vi "FileTrcOpen.vi"(6 "提示语":refnum<vi>, 7 "Language":u32, 8 "进度条":refnum<vi>, 9 "进度数值":refnum<vi>, 10 "报文行数统计":refnum<vi>, 11 "file path (dialog if empty)":path caption="文件路径 （空时为对话框）") -> (0 "路径输出":path, 1 "重构的Data数组":u32[][](array[numeric]), 2 "统计数量":string[](array[string]), 3 "报文ID":string[](array[string]), 4 "基时间簇":T1 {"基时间秒" format="%#.6f"}, 5 "CAN报文统计":string[][](array[string]))   [LabVIEW 2015]
uses:
  <vilib>/Utility/file.llb/Read Delimited Spreadsheet (string).vi
  <vilib>/regexp/Match Regular Expression.xnode
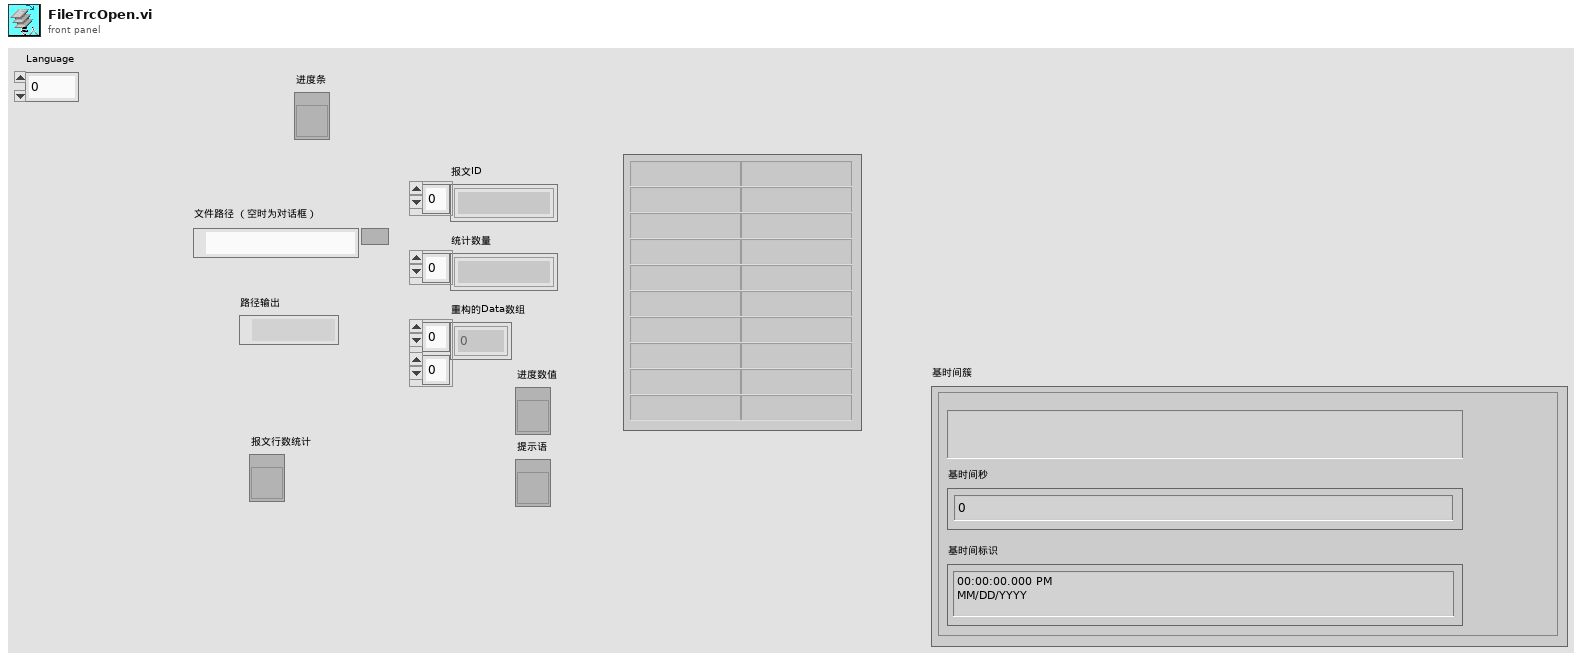
[diagram p1: front panel]
types:
  T1 = cluster{"基时间字符串":string, "基时间秒":dbl, "基时间标识":timestamp}
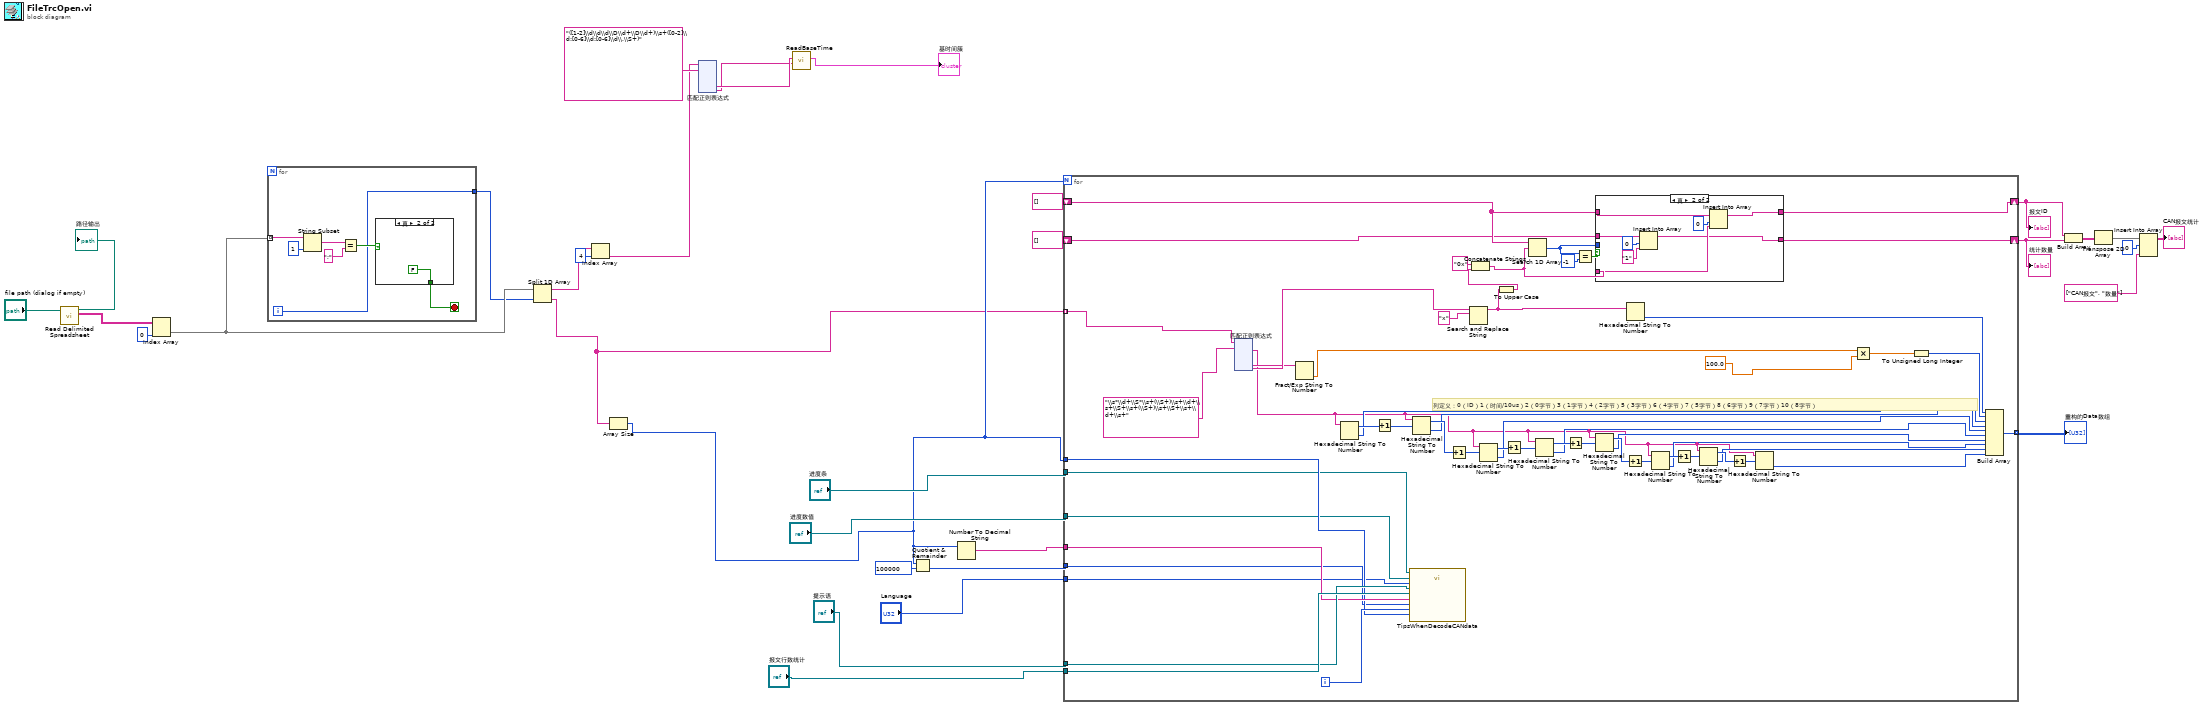
[diagram p0: block diagram]
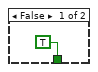
[diagram p2: hidden frame]
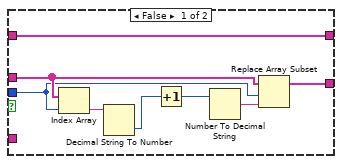
[diagram p3: hidden frame]
diagram:
  n1 = call-poly <vilib>:"Read Delimited Spreadsheet.vi"("file path (dialog if empty)"="file path (dialog if empty)") -> ("new file path (Not A Path if cancelled)"=→"路径输出":path, "all rows"=w12:string[][])  [unwired: 9 in, 4 out]
  n2 = Index Array(array=w12, index (col)=0 ("禁用的索引 (列)")) -> (element=w2:string[])  [unwired: 1 in]
  n3 = for {
    tunnel: w2 -> [w40] mode=indexing
    tunnel: [w34] -> w1
    i -> [w34]
    stop <- w35 stop-if-true
    n4 = String Subset(string=w40, length (rest)=1 ("长度（剩余）")) -> (substring=w38:string)  [unwired: 1 in]
    n5 = Equal?(x=w38, y=";") -> (x = y?=w36:bool)
    n6 = case shown="真" w36 {
      tunnel: [TRUE FALSE] -> w35
      frame False {
      }
      frame True {
      }
    }
  }
  n7 = Split 1D Array(array=w2, index=w1) -> (first subarray=w9:string[], second subarray=w8:string[])
  n8 = Index Array(array=w9, index=4 ("索引")) -> (element=w6:string)
  n9 = Array Size(array=w8) -> (size(s)=w11:i32)
  n10 = xnode "匹配正则表达式"("输入字符串"=w6, "正则表达式"="([1-2]\\d\\d\\d\\D\\d+\\D\\d+)\\s+([0-2]\\d:[0-6]\\d:[0-6]\\d\\.\\S+)") -> ("子匹配 1"=w5:string, "子匹配 2"=w4:string)  [unwired: 4 in, 5 out]
  n11 = call "ReadBaseTime.vi"("时间字符"=w4, "日期字符"=w5) -> ("基时间簇"=→"基时间簇":T1)  [unwired: 7 in]
  n12 = Quotient & Remainder(x=w11, y=100000) -> (floor(x/y)=w18:i32)  [unwired: 1 out]
  n13 = Number To Decimal String(number=w11) -> (decimal integer string=w16:string)  [unwired: 1 in]
  n14 = for {
    N: w11 -> [_]
    tunnel: [w74] -> w33 mode=indexing
    shift-right: [w70] -> w26
    shift-left: string[] [] -> [w71]
    shift-right: [w65] -> w25
    shift-left: string[] [] -> [w66]
    tunnel: w11 -> [w53]
    tunnel: "进度条" -> [w49]
    tunnel: "进度数值" -> [w50]
    tunnel: w18 -> [w52]
    tunnel: "提示语" -> [w55]
    tunnel: w16 -> [w54]
    tunnel: "报文行数统计" -> [w56]
    tunnel: "Language" -> [w51]
    tunnel: w8 -> [w48] mode=indexing
    i -> [w57]
    # "列定义：0（ID）1（时间/10us）2（0字节）3（1字节）4（2字节）5（3字节）6（4字节）7（5字节）8（6字节）9（7字节）10（8字节）"
    n15 = xnode "匹配正则表达式"("输入字符串"=w48, "正则表达式"="\\s*\\d+\\S*\\s+(\\S+)\\s+\\d+\\s+\\S+\\s+(\\S+)\\s+\\S+\\s+\\d+\\s+" ("格式字符串")) -> ("匹配之后"=w45:string, "子匹配 1"=w46:string, "子匹配 2"=w47:string)  [unwired: 4 in, 4 out]
    n16 = Fract/Exp String To Number(string=w46) -> (number=w44:dbl)  [unwired: 3 in, 1 out]
    n17 = Hexadecimal String To Number(string=w45) -> (offset past number=w95:i32, number=w82:u32)  [unwired: 2 in]
    n18 = Increment(x=w95) -> (x+1=w96:i32)
    n19 = call "TipsWhenDecodeCANdata.vi"("ProgressBar"=w49, "AllRowsNum"=w53, "i"=w57, "ProgressNum"=w50, "Language"=w51, "Tips"=w55, "MessageLinCnt"=w56, "txtAllRowsNum"=w54, "RowsLevel"=w52) -> ()  [unwired: 7 in]
    n20 = Hexadecimal String To Number(string=w45, offset=w96) -> (offset past number=w91:i32, number=w81:u32)  [unwired: 1 in]
    n21 = Increment(x=w91) -> (x+1=w92:i32)
    n22 = Search and Replace String(input string=w47, search string="x" ("子字符串(\"\")")) -> (result string=w60:string)  [unwired: 6 in, 3 out]
    n23 = Hexadecimal String To Number(string=w45, offset=w92) -> (offset past number=w94:i32, number=w80:u32)  [unwired: 1 in]
    n24 = To Upper Case(1:w60) -> (0:w61:string)
    n25 = Concatenate Strings("0x" ("字符串"), w61) -> (w62:string)
    n26 = Increment(x=w94) -> (x+1=w93:i32)
    n27 = Search 1D Array(1D array=w71, element=w62) -> (index of element=w64:i32)  [unwired: 1 in]
    n28 = Hexadecimal String To Number(string=w45, offset=w93) -> (offset past number=w83:i32, number=w79:u32)  [unwired: 1 in]
    n29 = Increment(x=w83) -> (x+1=w84:i32)
    n30 = Equal?(x=w64, y=-1) -> (x = y?=w68:bool)
    n31 = case shown="真" w68 {
      tunnel: w71 -> [w221 w229]
      tunnel: [w221 w228] -> w70
      tunnel: w62 -> [_ w227]
      tunnel: w66 -> [w220 w224]
      tunnel: [w219 w225] -> w65
      tunnel: w64 -> [w214 _]
      frame False {
        n32 = Index Array(array=w220, index=w214) -> (element=w218:string)
        n33 = Decimal String To Number(string=w218) -> (number=w217:i32)  [unwired: 2 in, 1 out]
        n34 = Increment(x=w217) -> (x+1=w215:i32)
        n35 = Number To Decimal String(number=w215) -> (decimal integer string=w216:string)  [unwired: 1 in]
        n36 = Replace Array Subset(array=w220, new element=w216, index=w214) -> (w219:string[])
      }
      frame True {
        n37 = Insert Into Array(array=w224, index=0 ("索引"), new element="1" ("新元素/子数组")) -> (w225:string[])
        n38 = Insert Into Array(array=w229, index=0 ("索引"), new element=w227) -> (w228:string[])
      }
    }
    n39 = Hexadecimal String To Number(string=w45, offset=w84) -> (offset past number=w86:i32, number=w78:u32)  [unwired: 1 in]
    n40 = Hexadecimal String To Number(string=w60) -> (number=w67:u32)  [unwired: 2 in, 1 out]
    n41 = Increment(x=w86) -> (x+1=w85:i32)
    n42 = Hexadecimal String To Number(string=w45, offset=w85) -> (offset past number=w90:i32, number=w77:u32)  [unwired: 1 in]
    n43 = Increment(x=w90) -> (x+1=w89:i32)
    n44 = Hexadecimal String To Number(string=w45, offset=w89) -> (offset past number=w87:i32, number=w76:u32)  [unwired: 1 in]
    n45 = Increment(x=w87) -> (x+1=w88:i32)
    n46 = Hexadecimal String To Number(string=w45, offset=w88) -> (number=w75:u32)  [unwired: 1 in, 1 out]
    n47 = Multiply(x=w44, y=100.0) -> (x*y=w73:dbl)
    n48 = To Unsigned Long Integer(number=w73) -> (unsigned 32bit integer=w72:u32)
    n49 = Build Array(w67, w72, w82, w81, w80, w79, w78, w77, w76, w75) -> (w74:u32[])
  }
  "重构的Data数组" <- w33
  "报文ID" <- w26
  "统计数量" <- w25
  n50 = Build Array(w26, w25) -> (w30:string[][])
  n51 = Transpose 2D Array(2D array=w30) -> (transposed array=w29:string[][])
  n52 = Insert Into Array(array=w29, index (row)=0 ("索引 (行)"), new element=string[] ["CAN报文", "数量"]) -> (→"CAN报文统计":string[][])  [unwired: 1 in]
